vi "Black Box File Convert.vi"(3 "Path":path) -> ()   [LabVIEW 2022 SP3]
panel:
  out "resulting string":string
  out "Channel":string
  out "ESN":string
  out "appended array":string[][](array[string])
  out "New Filename":string
  out "array":string[][](array[string])
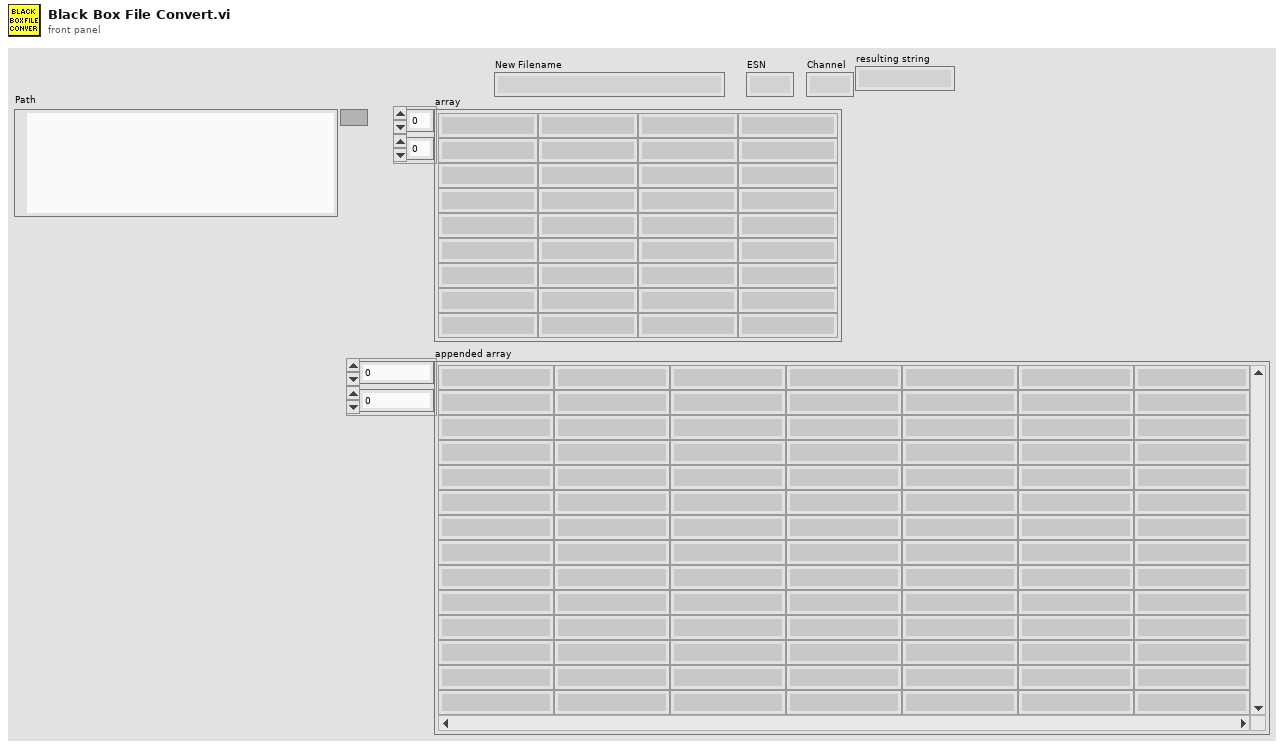
[diagram p1: front panel]
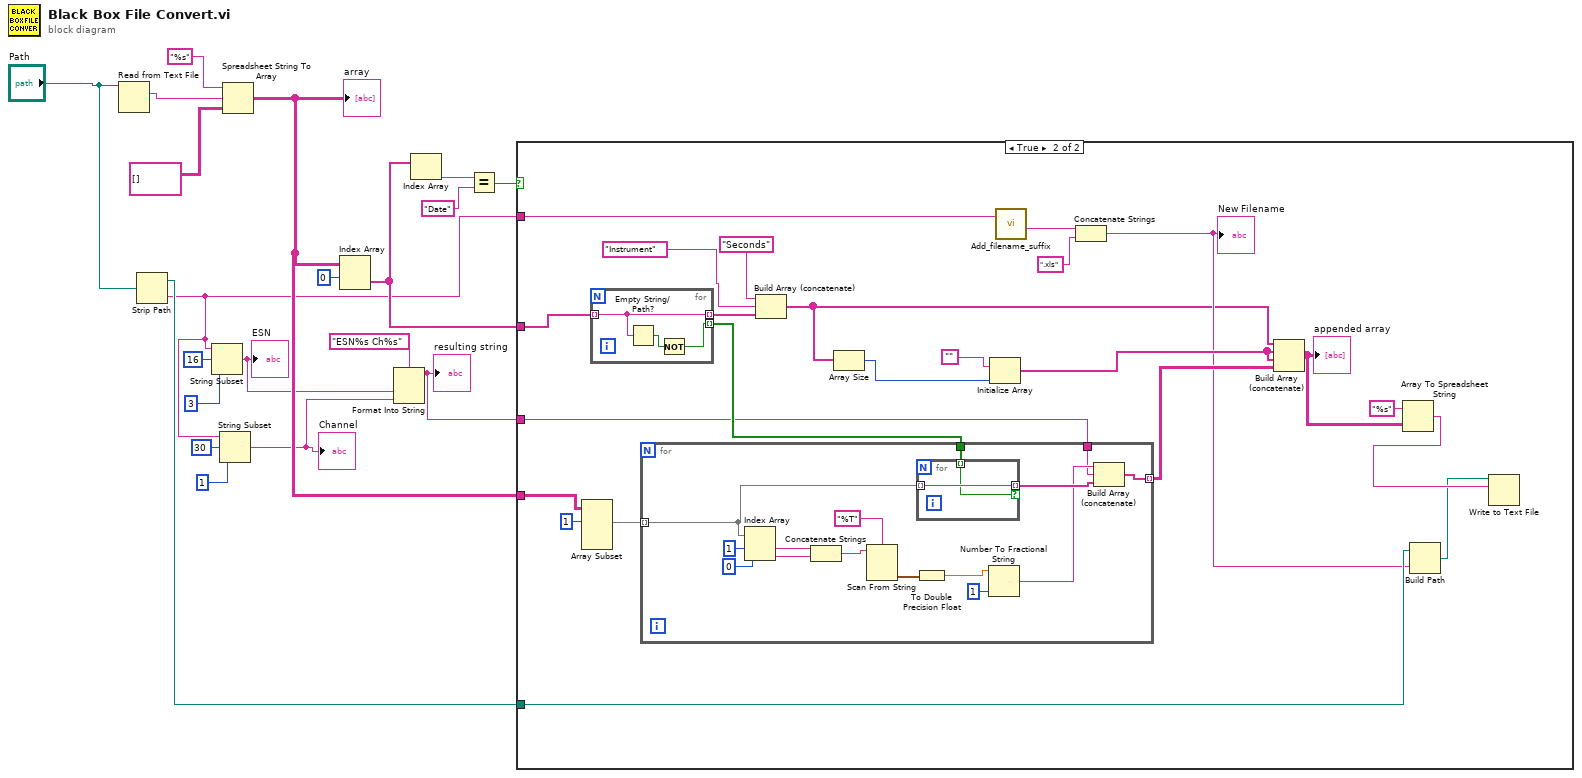
[diagram p0: block diagram]
diagram:
  n1 = Read from Text File(file (use dialog)="Path") -> (text=w20:string)  [unwired: 3 in, 3 out]
  n2 = Strip Path(path="Path") -> (stripped path=w10:path, name=w7:string)
  n3 = String Subset(string=w7, offset (0)=16, length (rest)=3 ("length (rest)")) -> (substring=w4:string)
  "ESN" <- w4
  n4 = String Subset(string=w7, offset (0)=30, length (rest)=1 ("length (rest)")) -> (substring=w3:string)
  "Channel" <- w3
  n5 = Spreadsheet String To Array(format string="%s", spreadsheet string=w20, array type (2D Dbl)=string[][] []) -> (array=w11:string[][])  [unwired: 1 in]
  "array" <- w11
  n6 = Index Array(array=w11, index (row)=0) -> (element=w16:string[])  [unwired: 1 in]
  n7 = Format Into String(format string="ESN%s Ch%s", w4, w3) -> (resulting string=w1:string)  [unwired: 2 in, 1 out]
  "resulting string" <- w1
  n8 = Index Array(array=w16) -> (element=w15:string)  [unwired: 1 in]
  n9 = Equal?(x=w15, y="Date") -> (x = y?=w13:bool)
  n10 = case shown="True" w13 {
    tunnel: w16 -> [_ w27]
    tunnel: w7 -> [_ w37]
    tunnel: w11 -> [_ w36]
    tunnel: w10 -> [_ w30]
    tunnel: w1 -> [_ w21]
    frame False {
    }
    frame True {
      n11 = Array Subset(array=w36, index (row)=1 ("index")) -> (w42:string[][])  [unwired: 3 in]
      n12 = for {
        tunnel: [w45] -> w26 mode=indexing if=w44
        tunnel: w27 -> [w45] mode=indexing
        tunnel: [w44] -> w25 mode=indexing
        n13 = Empty String/Path?(string/path=w45) -> (empty?=w46:bool)
        n14 = Not(x=w46) -> (.not. x?=w44:bool)
      }
      n15 = for {
        tunnel: w42 -> [w50] mode=indexing
        tunnel: [w52] -> w41 mode=indexing
        tunnel: w25 -> [w49]
        tunnel: w21 -> [w47]
        n16 = Index Array(array=w50, index #1=1 ("index"), index #2=0 ("index")) -> (element #1=w60:string, element #2=w61:string)
        n17 = Concatenate Strings(w60, w61) -> (w57:string)
        n18 = Scan From String(format string="%T", input string=w57) -> (output 1=w58:timestamp)  [unwired: 3 in, 3 out]
        n19 = for {
          tunnel: [w63] -> w51 mode=indexing if=w62
          tunnel: w50 -> [w63] mode=indexing
          tunnel: w49 -> [w62] mode=indexing
        }
        n20 = To Double Precision Float(number=w58) -> (double precision float=w59:dbl)
        n21 = Number To Fractional String(number=w59, precision (6)=i16 1) -> (F-format string=w48:string)  [unwired: 2 in]
        n22 = Build Array (concatenate)(w48, w47, w51) -> (w52:string[])
      }
      n23 = Build Array (concatenate)("Seconds", "Instrument", w26) -> (w24:string[])
      n24 = Array Size(array=w24) -> (size(s)=w40:i32)
      n25 = Initialize Array("", w40) -> (w38:string[])
      n26 = call "Add_filename_suffix.vi"("Filename"=w37) -> ("Base name"=w34:string)  [unwired: 1 in, 3 out]
      n27 = Concatenate Strings(w34, ".xls" ("Suffix to add")) -> (w29:string)
      "New Filename" <- w29
      n28 = Build Array (concatenate)(w24, w38, w38, w41) -> (w33:string[][])
      "appended array" <- w33
      n29 = Array To Spreadsheet String(array=w33, 3:"%s" ("format string")) -> (spreadsheet string=w31:string)  [unwired: 1 in]
      n30 = Build Path(base path=w30, name or relative path=w29) -> (appended path=w28:path)
      n31 = Write to Text File(file (use dialog)=w28, text=w31) -> ()  [unwired: 2 in, 3 out]
    }
  }
